vi "CF_FP to PGSQL.vi"(8 "error in (no error)":errorcluster, 10 "str":string[](array[string]), 11 "dbl":dbl[](array[numeric])) -> (0 "error out":errorcluster)   [LabVIEW 2013]
uses:
  shared/postgreSQL-lv/Data.PG/Data.PGSQL.lvclass
panel:
  # "CF FP to PGSQL"
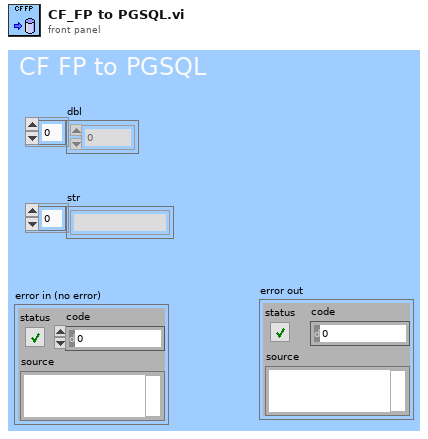
[diagram p1: front panel]
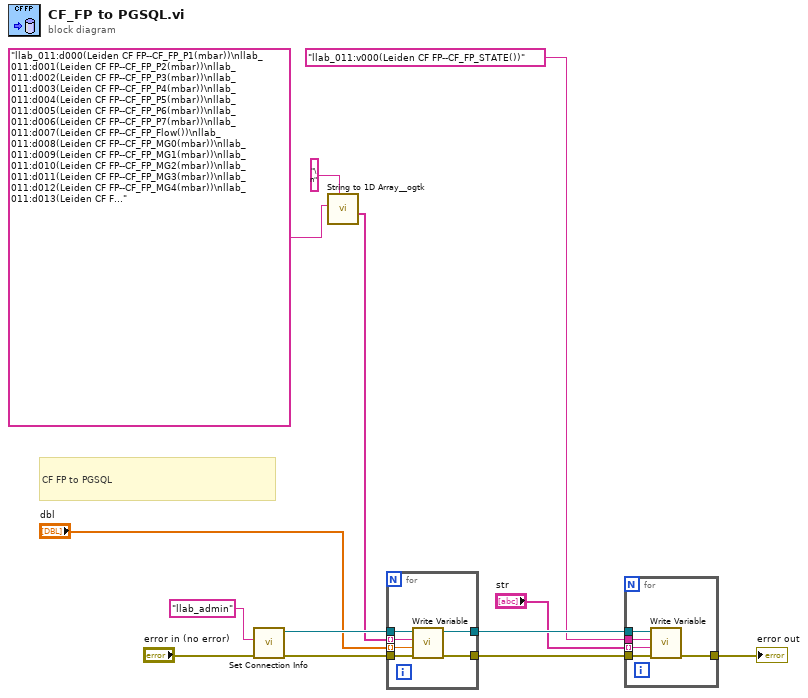
[diagram p0: block diagram]
diagram:
  # "CF FP to PGSQL"
  n1 = call "Set Connection Info.vi"("username"="llab_admin", "error in (no error)"="error in (no error)") -> ("Data.PG out"=w12:refnum<class "Data.PGSQL.lvclass">, "error out"=w13:errorcluster)  [unwired: 7 in]
  n2 = call <userlib>:"String to 1D Array__ogtk.vi"("delimiter (Tab)"="\n", "string"="llab_011:d000(Leiden CF FP--CF_FP_P1(mbar))\nllab_011:d001(Leiden CF FP--CF_FP_P2(mbar))\nllab_011:d002(Leiden CF FP--CF_FP_P3(mbar))\nllab_011:d003(Leiden CF FP--CF_FP_P4(mbar))\nllab_011:d004(Leiden CF FP--CF_FP_P5(mbar))\nllab_011:d005(Leiden CF FP--CF_FP_P6(mbar))\nllab_011:d006(Leiden CF FP--CF_FP_P7(mbar))\nllab_011:d007(Leiden CF FP--CF_FP_Flow())\nllab_011:d008(Leiden CF FP--CF_FP_MG0(mbar))\nllab_011:d009(Leiden CF FP--CF_FP_MG1(mbar))\nllab_011:d010(Leiden CF FP--CF_FP_MG2(mbar))\nllab_011:d011(Leiden CF FP--CF_FP_MG3(mbar))\nllab_011:d012(Leiden CF FP--CF_FP_MG4(mbar))\nllab_011:d013(Leiden CF FP--CF_FP_MG5(mbar))\nllab_011:d014(Leiden CF FP--CF_FP_PT_on())\nllab_011:d015(Leiden CF FP--CF_FP_PT_W_in_T(K))\nllab_011:d016(Leiden CF FP--CF_FP_PT_W_out_T(K))\nllab_011:d017(Leiden CF FP--CF_FP_PT_He_T(K))\nllab_011:d018(Leiden CF FP--CF_FP_PT_oil_T(K))\nllab_011:d019(Leiden CF FP--CF_FP_PT_P_Low(bar))\nllab_011:d020(Leiden CF FP--CF_FP_PT_P_High(bar))\nllab_011:d021(Leiden CF FP--CF_FP_PT_current(A))\nllab_011:d022(Leiden CF FP--CF_FP_state0())\nllab_011:d023(Leiden CF FP--CF_FP_state1())\nllab_011:d024(Leiden CF FP--CF_FP_state2())") -> ("Array of Strings"=w4:string[])  [unwired: 9 in]
  n3 = for {
    tunnel: w13 -> [w19]
    tunnel: w12 -> [w18]
    tunnel: w4 -> [w17] mode=indexing
    tunnel: [w16] -> w9
    tunnel: [w15] -> w8
    tunnel: "dbl" -> [w14] mode=indexing
    n4 = call "Write Variable.vi"("error in (no error)"=w19, "Data"=w14, "variable"=w17, "Data.PG in"=w18) -> ("error out"=w16:errorcluster, "Data.PG out"=w15:refnum<class "Data.PGSQL.lvclass">)  [unwired: 5 in, 1 out]
  }
  n5 = for {
    tunnel: w9 -> [w24]
    tunnel: w8 -> [w23]
    tunnel: [w22] -> w7
    tunnel: "llab_011:v000(Leiden CF FP--CF_FP_STATE())" -> [w21]
    tunnel: "str" -> [w20] mode=indexing
    n6 = call "Write Variable.vi"("error in (no error)"=w24, "Data"=w20, "variable"=w21, "Data.PG in"=w23) -> ("error out"=w22:errorcluster)  [unwired: 5 in, 2 out]
  }
  "error out" <- w7
